vi "GeoFonu_v1.5.vi"() -> ()   [LabVIEW 2014]
uses:
  <vilib>/Instr/_visa.llb/VISA Set IO Buffer Mask.ctl
  <vilib>/Instr/_visa.llb/VISA Flush IO Buffer Mask.ctl
  <vilib>/Instr/_visa.llb/VISA Configure Serial Port (Instr).vi
panel:
  out "Real time":timestamp
  out "Sensor3":i32[](graph)
  out "Sensor2":i32[](graph)
  out "Sensor1":i32[](graph)
  in  "milliseconds to wait":u32=500
  in  "stop":bool
  in  "VISA resource name":refnum<visa-resource-name>
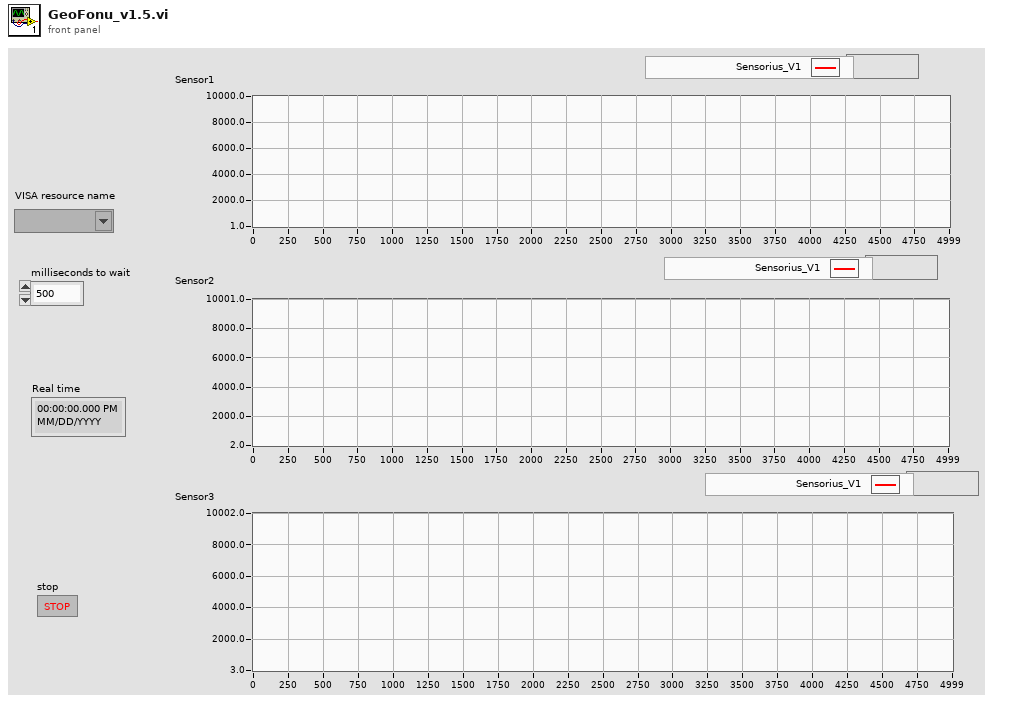
[diagram p1: front panel]
types:
  T1 = typedef "VISA Set IO Buffer Mask.ctl" = u16
  T2 = typedef "VISA Flush IO Buffer Mask.ctl" = u16
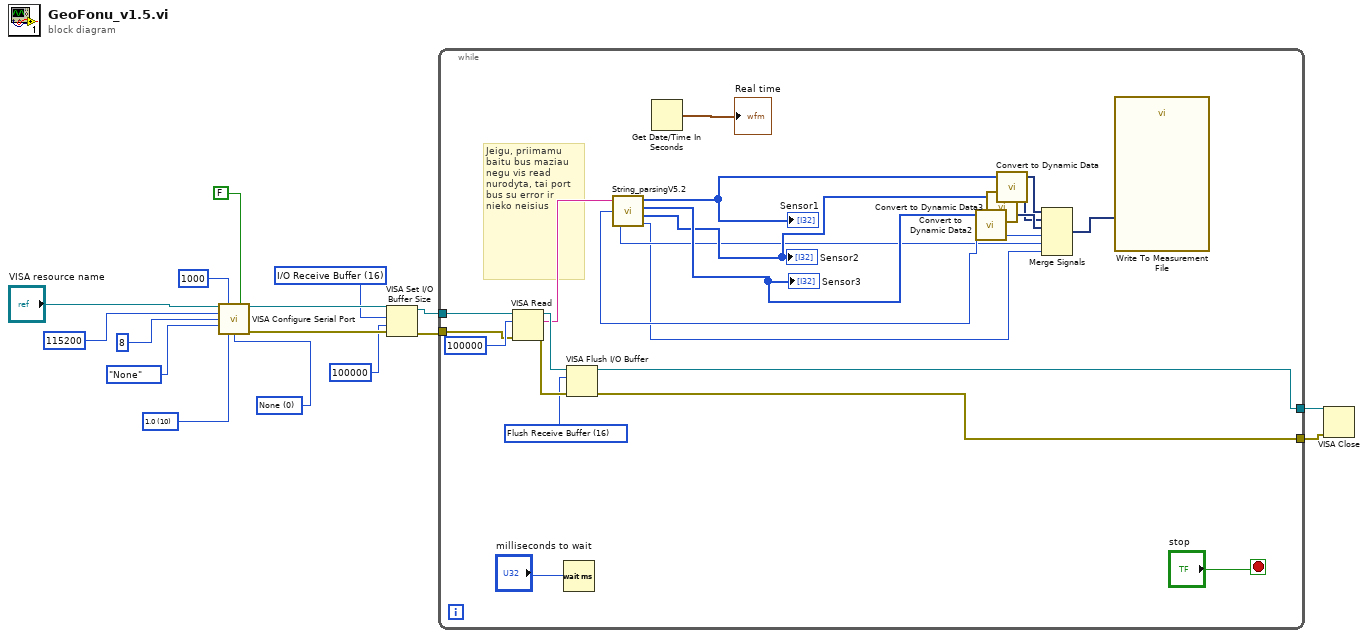
[diagram p0: block diagram]
diagram:
  w6 = T1 16 items=["I/O Receive Buffer"=16, "I/O Transmit Buffer"=32, "I/O Receive and Transmit Buffer"=48] ("Mask")
  w12 = u16 0 items=["None", "XON/XOFF", "RTS/CTS", "XON/XOFF & RTS/CTS", "DTR/DSR", "XON/XOFF & DTR/DSR"] ("flow control (0:none)")
  w13 = u16 10 items=["1.0"=10, "1.5"=15, "2.0"=20] ("stop bits (10: 1 bit)")
  n1 = call-poly "VISA Configure Serial Port"("VISA resource name"="VISA resource name", "timeout (10sec)"=u32 1000, "Enable Termination\nChar (T)"=FALSE ("Enable Termination\nChar (T)"), "baud rate (9600)"=u32 115200, "data bits (8)"=u16 8, "parity (0:none)"=enum16{"None", "Odd", "Even", "Mark", "Space"}."None", "stop bits (10: 1 bit)"=w13, "flow control (0:none)"=w12) -> ("VISA resource name out"=w8:refnum<visa-resource-name>, "error out"=w9:errorcluster)  [unwired: 6 in]
  n2 = VISA Set I/O Buffer Size(VISA resource name=w8, mask (16)=w6, size (4096)=u32 100000, error in (no error)=w9) -> (VISA resource name out=w3:refnum<visa-resource-name>, error out=w5:errorcluster)
  n3 = while {
    tunnel: w3 -> [w38]
    tunnel: w5 -> [w35]
    tunnel: [w30] -> w2
    tunnel: [w29] -> w1
    stop <- "stop" stop-if-true
    w32 = T2 16 items=["Flush Receive Buffer"=16, "Write Transmit Buffer to Device"=32, "Flush Receive Buffer (No I/O)"=64, "Flush Transmit Buffer"=128] ("Mask")
    # "Jeigu, priimamu baitu bus maziau negu vis read nurodyta, tai port bus su error ir nieko neisius"
    n4 = VISA Read(VISA resource name=w38, byte count=u32 100000, error in (no error)=w35) -> (VISA resource name out=w34:refnum<visa-resource-name>, read buffer=w24:string, error out=w33:errorcluster)  [unwired: 1 out]
    n5 = Wait (ms)(milliseconds to wait="milliseconds to wait") -> ()  [unwired: 1 out]
    n6 = VISA Flush I/O Buffer(VISA resource name=w34, mask (16)=w32, error in (no error)=w33) -> (VISA resource name out=w30:refnum<visa-resource-name>, error out=w29:errorcluster)
    n7 = call "String_parsingV5.2.vi"("input string"=w24) -> ("sekundes"=w20:i32, "minute"=w19:i32, "V1"=w23:i32[], "V3"=w22:i32[], "V2"=w21:i32[], "hour"=w18:i32)
    "Sensor1" <- w23
    "Sensor2" <- w21
    "Sensor3" <- w22
    n8 = Get Date/Time In Seconds() -> (seconds since 1Jan1904=→"Real time":timestamp)
    n9 = call "Convert to Dynamic Data2"("Array"=w22) -> ("Dynamic Data Type"=w26:dynamicdata)  [unwired: 3 in]
    n10 = call "Convert to Dynamic Data3"("Array"=w21) -> ("Dynamic Data Type"=w25:dynamicdata)  [unwired: 3 in]
    n11 = call "Convert to Dynamic Data"("Array"=w23) -> ("Dynamic Data Type"=w28:dynamicdata)  [unwired: 3 in]
    n12 = Merge Signals(w28, w25, w26, w20, w19, w18) -> (w27:dynamicdata)
    n13 = call "Write To Measurement File"("Signals"=w27) -> ()  [unwired: 16 in, 3 out]
  }
  n14 = VISA Close(VISA resource name=w2, error in (no error)=w1) -> ()  [unwired: 1 out]
